vi "AC concatentated string command.vi"(9 "DesignRequest":T1, 10 "AC Variables":string[](array[string]), 11 "MathCAD results":T2) -> (1 "MathCAD AC":T2, 2 "Has AC commands":bool, 3 "AC concatenated string":string)   [LabVIEW 2012, in "Design Server.lvlib"]
uses:
  Design Server.lvlib
  Variable cluster.ctl
  Design Request.ctl
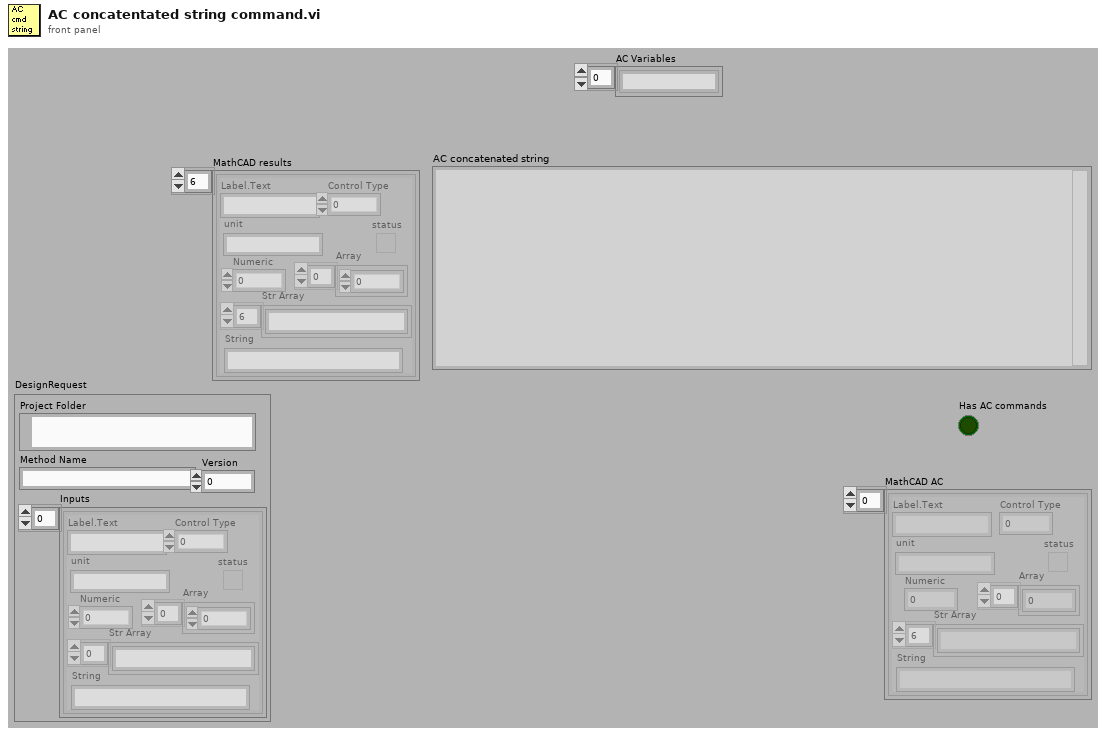
[diagram p1: front panel]
types:
  T1 = typedef "Design Server.lvlib/Design Request.ctl" = cluster{"Project Folder":path, "Method Name":string, "Inputs":T2, "Version":i32}
  T2 = typedef "Design Server.lvlib/Variable cluster.ctl" = cluster{"Label.Text":string, "Control Type":u32, "Numeric":dbl, "Array":dbl[], "status":bool, "Str Array":string[], "String":string, "unit":string}[]
  T3 = cluster{"index of element":i32, "output cluster":cluster{"Label.Text":string, "Control Type":u32, "Numeric":dbl, "Array":dbl[], "status":bool, "Str Array":string[], "String":string, "unit":string}}[]
  T4 = cluster{"index of element":i32, "output cluster":cluster{"Label.Text":string, "Control Type":u32, "Numeric":dbl, "Array":dbl[], "status":bool, "Str Array":string[], "String":string, "unit":string}}
  T5 = cluster{"Label.Text":string, "Control Type":u32, "Numeric":dbl, "Array":dbl[], "status":bool, "Str Array":string[], "String":string, "unit":string}
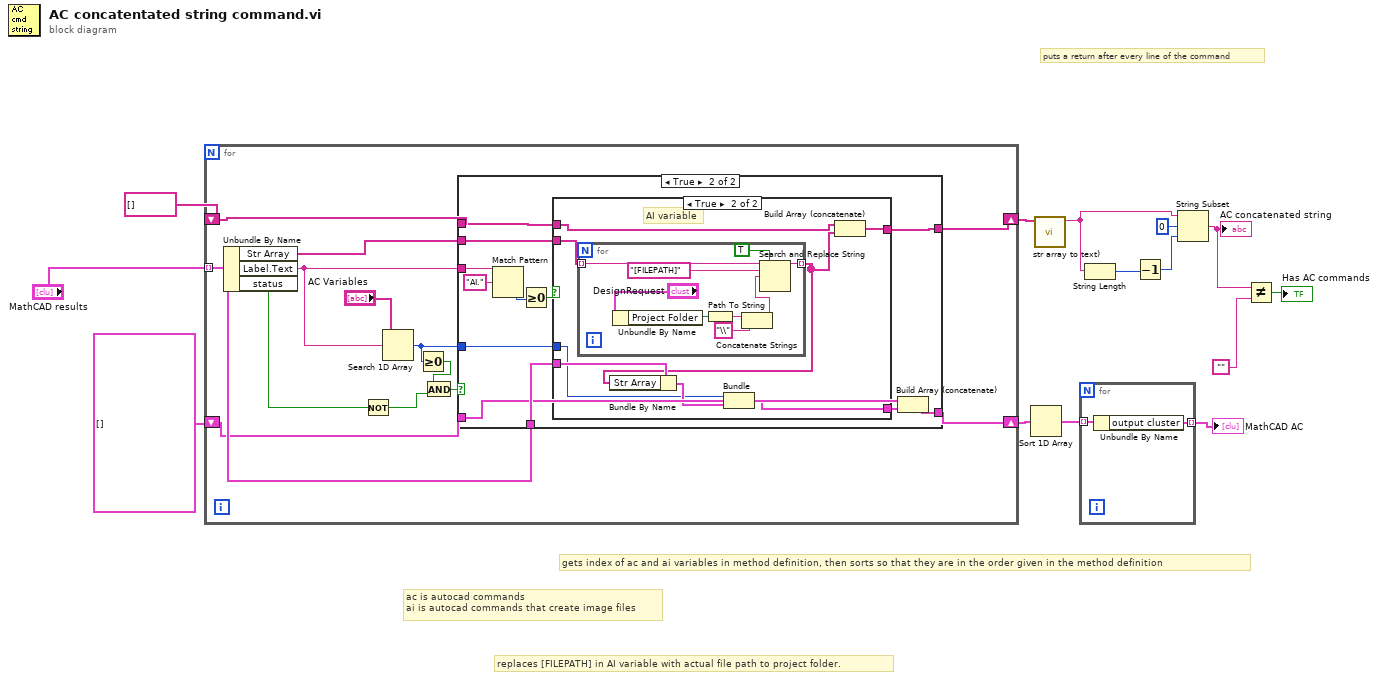
[diagram p0: block diagram]
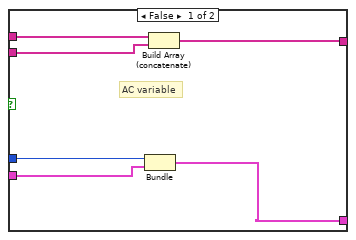
[diagram p3: hidden frame]
diagram:
  # "replaces [FILEPATH] in AI variable with actual file path to project folder."
  # "ac is autocad commands\nai is autocad commands that create image files"
  # "gets index of ac and ai variables in method definition, then sorts so that they are in the order given in the method definition"
  # "puts a return after every line of the command"
  n1 = for {
    tunnel: "MathCAD results" -> [w21] mode=indexing
    shift-right: [w27] -> w9
    shift-left: string[] [] -> [w26]
    shift-right: [w20] -> w5
    shift-left: T3 [] -> [w19]
    n2 = Unbundle By Name(w21) -> ("Str Array"=w22:string[], "Label.Text"=w15:string, "status"=w25:bool)
    n3 = Not(x=w25) -> (.not. x?=w24:bool)
    n4 = Search 1D Array(1D array="AC Variables", element=w15) -> (index of element=w16:i32)  [unwired: 1 in]
    n5 = Greater Or Equal To 0?(x=w16) -> (x >= 0?=w17:bool)
    n6 = And(x=w17, y=w24) -> (x .and. y?=w23:bool)
    n7 = case shown="True" w23 {
      tunnel: [w29 w30] -> w27
      tunnel: w26 -> [w29 w41]
      tunnel: w22 -> [_ w40]
      tunnel: w21 -> [_ w37]
      tunnel: [w28 w39] -> w20
      tunnel: w19 -> [w28 w35]
      tunnel: w16 -> [_ w38]
      tunnel: w15 -> [_ w34]
      frame False {
      }
      frame True {
        n8 = Match Pattern(string=w34, regular expression="AI.") -> (offset past match=w32:i32)  [unwired: 1 in, 3 out]
        n9 = Greater Or Equal To 0?(x=w32) -> (x >= 0?=w31:bool)
        n10 = case shown="True" w31 {
          tunnel: [w47 w48] -> w30
          tunnel: w41 -> [w46 w50]
          tunnel: w40 -> [w45 w54]
          tunnel: w38 -> [w44 w52]
          tunnel: w37 -> [w43 w55]
          tunnel: [w42 w51] -> w36
          frame False {
            # "AC variable"
            n11 = Bundle("index of element"=w44, "output cluster"=w43) -> (w42:T4)  [unwired: 1 in]
            n12 = Build Array (concatenate)(w46, w45) -> (w47:string[])
          }
          frame True {
            # "AI variable"
            n13 = for {
              tunnel: w54 -> [w64] mode=indexing
              tunnel: [w62] -> w49 mode=indexing
              n14 = Unbundle By Name("DesignRequest") -> ("Project Folder"=w60:path)
              n15 = Path To String(path=w60) -> (string=w59:string)
              n16 = Concatenate Strings(w59, "\\" ("string")) -> (w58:string)
              n17 = Search and Replace String(replace all?=TRUE ("replace all? (F)"), input string=w64, search string="[FILEPATH]", replace string=w58) -> (result string=w62:string)  [unwired: 4 in, 3 out]
            }
            n18 = Bundle By Name(cluster=w55, "Str Array"=w49) -> (w53:T5)
            n19 = Bundle("index of element"=w52, "output cluster"=w53) -> (w51:T4)  [unwired: 1 in]
            n20 = Build Array (concatenate)(w50, w49) -> (w48:string[])
          }
        }
        n21 = Build Array (concatenate)(w35, w36) -> (w39:T3)
      }
    }
  }
  n22 = Sort 1D Array(array=w5) -> (sorted array=w4:T3)
  n23 = call "str array to text).vi"("Array"=w9) -> ("String"=w8:string)  [unwired: 10 in]
  n24 = for {
    tunnel: w4 -> [w66] mode=indexing
    tunnel: [w65] -> w2 mode=indexing
    n25 = Unbundle By Name(w66) -> ("output cluster"=w65:T5)
  }
  "MathCAD AC" <- w2
  n26 = String Length(string=w8) -> (length=w11:i32)
  n27 = Decrement(x=w11) -> (x-1=w10:i32)
  n28 = String Subset(string=w8, offset (0)=0, length (rest)=w10) -> (substring=w7:string)
  "AC concatenated string" <- w7
  n29 = Not Equal?(x=w7, y="") -> (x != y?=→"Has AC commands":bool)
